vi "Write To FPGA.vi"(7 "Group.Rate":u32[](array[numeric]), 8 "error in (no error)":errorcluster, 9 "Changed?":bool[](array[boolean]), 10 "Values":dbl[](array[numeric]), 11 "FPGA Refs":T1 {"Data Type" format="%.0x"}) -> (0 "error out":errorcluster, 2 "Values out":dbl[](array[numeric]), 3 "FPGA Refs":T1 {"Data Type" format="%.0x"})   [LabVIEW 2019, in "Fuel Injector Analysis Addon Engine.lvlib"]
uses:
  Fuel Injector Analysis Addon Engine.lvlib
  Types/FPGA Refs.ctl
  Addon Shared/Types/FPGA Data Types.ctl
  <vilib>/Utility/error.llb/Error Cluster From Error Code.vi
  <vilib>/rvi/errors/niLvFpgaAdjustHostInterfaceError.vi
  <vilib>/rvi/interface/nirviReadWriteControl/nirviReadWriteControl.xnode
  <vilib>/rvi/interface/Simulation/niFpgaSimulationCallBeginRW.vi
  NiFpgaLv.dll
  Addon Shared/Fuel Injector Analysis Addon Shared.lvlib
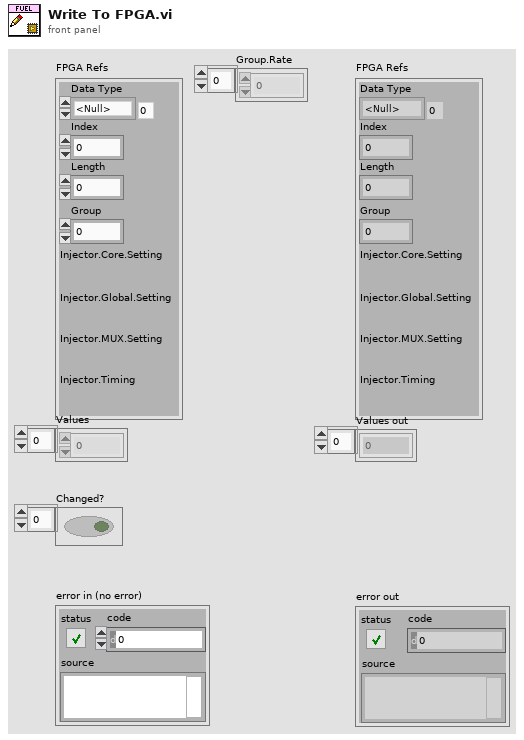
[diagram p1: front panel]
types:
  T1 = typedef "Fuel Injector Analysis Addon Engine.lvlib/FPGA Refs.ctl" = cluster{"Data Type":T2, "Index":i32, "Length":i32, "Group":i32, "Injector.Core.Setting":refnum<k20>, "Injector.Global.Setting":refnum<k20>, "Injector.MUX.Setting":refnum<k20>, "Injector.Timing":refnum<k20>}
  T2 = typedef "Fuel Injector Analysis Addon Shared.lvlib/FPGA Data Types.ctl" = enum8{"<Null>", "Injector.Core.Setting", "Injector.Global.Setting", "Injector.Mux.Setting", "Injector.Timing"}
  T3 = cluster{"Voltage Offset":fxp<+/-,32,8>, "Current Offset":fxp<+/-,32,8>}
  T4 = cluster{"Enable?":bool, "Initial Voltage Threshold":fxp<+/-,32,8>, "Event Dwell Limit":u16, "Voltage Gain":fxp<+/-,32,8>, "Current Gain":fxp<+/-,32,8>, "Filter Samples":u8, "Pretrigger Samples":u8, "Active Edge":bool}
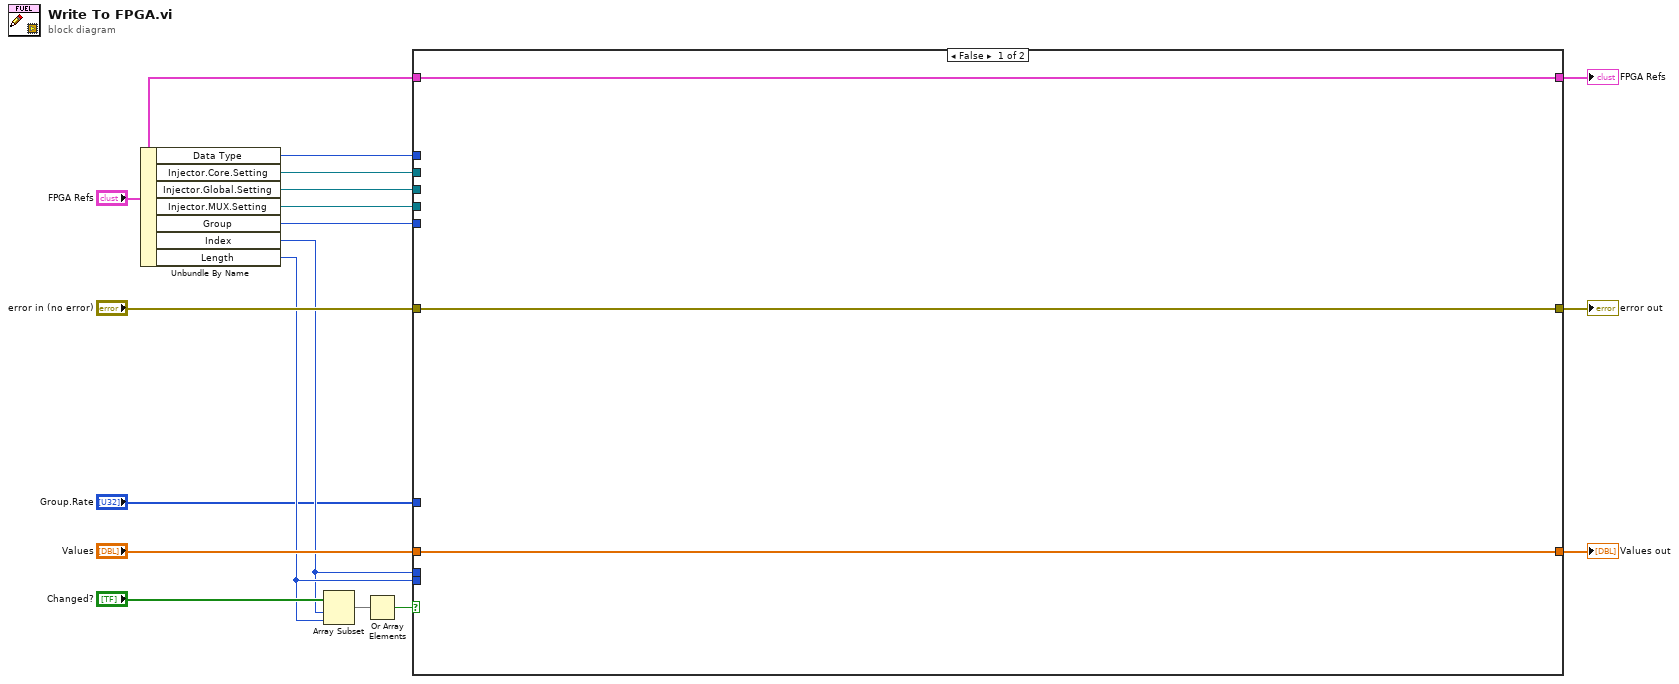
[diagram p0: block diagram]
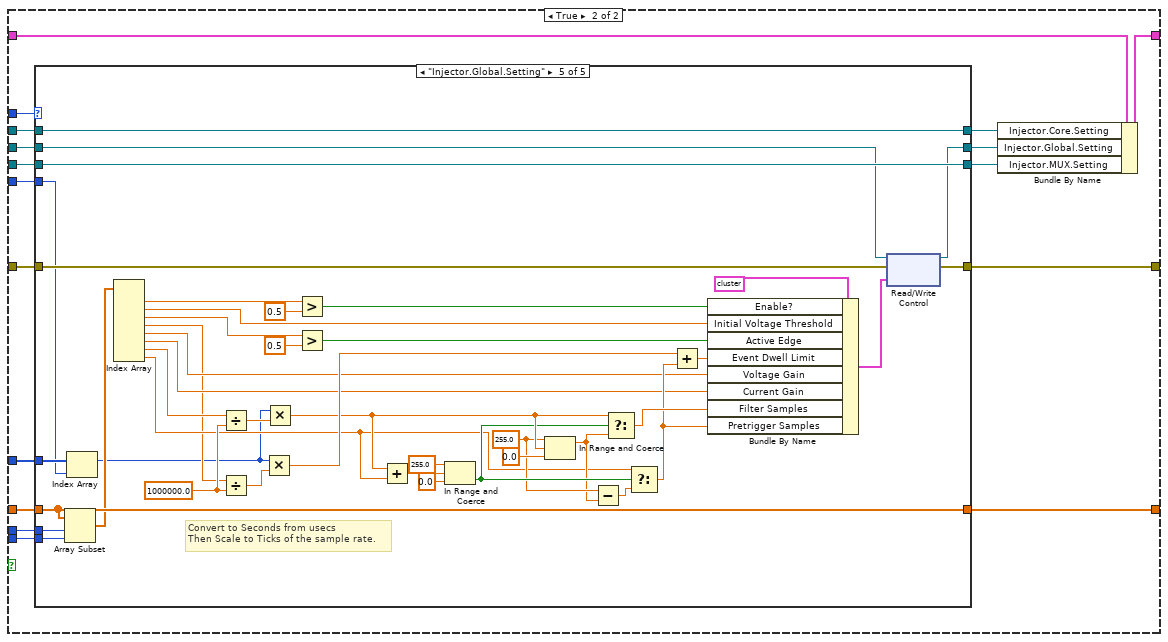
[diagram p2: hidden frame]
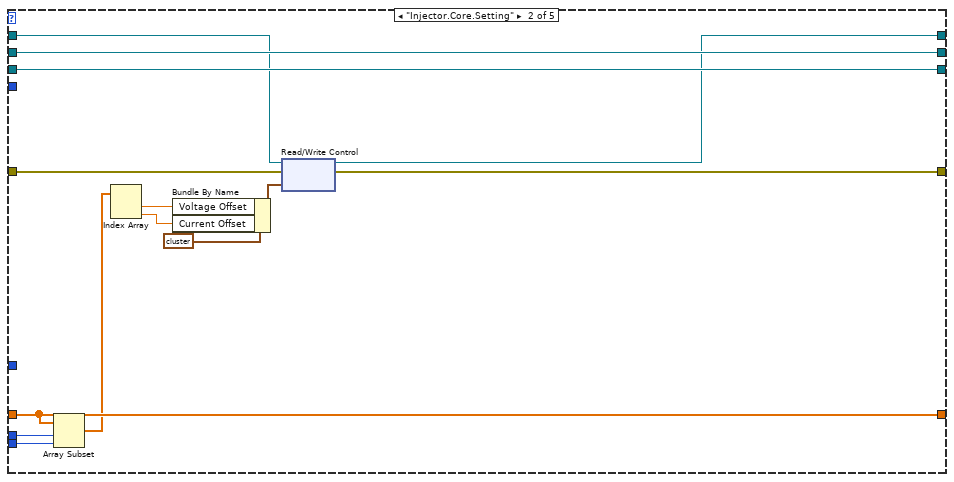
[diagram p4: hidden frame]
diagram:
  n1 = Unbundle By Name("FPGA Refs") -> ("Data Type"=w17:T2, "Injector.Core.Setting"=w8:refnum<k20>, "Injector.Global.Setting"=w12:refnum<k20>, "Injector.MUX.Setting"=w13:refnum<k20>, "Group"=w1:i32, "Index"=w3:i32, "Length"=w4:i32)
  n2 = Array Subset(array="Changed?", index=w3, length=w4) -> (w10:bool[])
  n3 = Or Array Elements(Boolean array=w10) -> (logical OR=w9:bool)
  n4 = case shown="False" w9 {
    tunnel: w17 -> [_ w37]
    tunnel: "error in (no error)" -> [w19 w36]
    tunnel: [w19 w35] -> w16
    tunnel: "FPGA Refs" -> [w20 w34]
    tunnel: [w20 w33] -> w5
    tunnel: [w18 w32] -> w15
    tunnel: "Values" -> [w18 w31]
    tunnel: w13 -> [_ w30]
    tunnel: w12 -> [_ w27]
    tunnel: w3 -> [_ w26]
    tunnel: w4 -> [_ w25]
    tunnel: w8 -> [_ w24]
    tunnel: "Group.Rate" -> [_ w22]
    tunnel: w1 -> [_ w21]
    frame False {
    }
    frame True {
      n5 = case shown="\"Injector.Global.Setting\"" w37 {
        tunnel: w36 -> [w42 w55 w59 w64 w109]
        tunnel: [w42 w54 w59 w64 w108] -> w35
        tunnel: [w41 w51 w60 w65 w105] -> w32
        tunnel: w31 -> [w41 w51 w60 w65 w105]
        tunnel: w25 -> [_ w52 _ _ w106]
        tunnel: w26 -> [_ w53 _ _ w107]
        tunnel: w30 -> [w40 w49 w57 w62 w103]
        tunnel: [w40 w49 w57 w62 w103] -> w29
        tunnel: [w39 w56 w61 w66 w98] -> w28
        tunnel: w27 -> [w39 w56 w61 w66 w99]
        tunnel: w24 -> [w38 w48 w58 w63 w100]
        tunnel: [w38 w47 w58 w63 w100] -> w23
        tunnel: w22 -> [_ _ _ _ w94]
        tunnel: w21 -> [_ _ _ _ w67]
        frame "<Null>", Default {
        }
        frame "Injector.Core.Setting" {
          n6 = Array Subset(array=w51, index=w53, length=w52) -> (w50:dbl[])
          n7 = Index Array(array=w50) -> (element #1=w44:dbl, element #2=w43:dbl)  [unwired: 2 in]
          n8 = Bundle By Name(cluster=T3 {"Voltage Offset"=0.0, "Current Offset"=0.0} ("Value"), "Voltage Offset"=w44, "Current Offset"=w43) -> (w45:T3)
          n9 = xnode "Read/Write Control"("FPGA VI Reference In"=w48, "error in"=w55, "Value"=w45) -> ("FPGA VI Reference Out"=w47:refnum<k20>, "error out"=w54:errorcluster)
        }
        frame "Injector.Mux.Setting" {
          # "DLE NOTE - Only Set in Init"
        }
        frame "Injector.Timing" {
          # "DLE NOTE - Only Set in Init"
        }
        frame "Injector.Global.Setting" {
          w82 = 255.0 ("upper limit")
          w93 = 1000000.0 ("y")
          # "Convert to Seconds from usecs\nThen Scale to Ticks of the sample rate."
          n10 = Array Subset(array=w105, index=w107, length=w106) -> (w104:dbl[])
          n11 = Index Array(array=w94, index=w67) -> (element=w68:u32)
          n12 = Index Array(array=w104) -> (element #1=w102:dbl, element #2=w101:dbl, element #3=w72:dbl, element #4=w74:dbl, element #5=w75:dbl, element #6=w76:dbl, element #7=w77:dbl, element #8=w78:dbl)  [unwired: 8 in]
          n13 = Divide(x=w77, y=w93) -> (x/y=w95:dbl)
          n14 = Divide(x=w74, y=w93) -> (x/y=w96:dbl)
          n15 = Multiply(x=w68, y=w96) -> (x*y=w88:dbl)
          n16 = Multiply(x=w68, y=w95) -> (x*y=w84:dbl)
          n17 = Greater?(x=w102, y=0.5 ("x")) -> (0:w71:bool)
          n18 = Greater?(x=w72, y=0.5 ("x")) -> (0:w70:bool)
          n19 = Add(x=w84, y=w78) -> (x+y=w92:dbl)
          n20 = In Range and Coerce(upper limit=255.0, x=w92, lower limit=0.0) -> (In Range?=w83:bool)  [unwired: 1 out]
          n21 = In Range and Coerce(upper limit=w82, x=w84, lower limit=0.0) -> (coerced(x)=w81:dbl)  [unwired: 1 out]
          n22 = Subtract(x=w82, y=w81) -> (x-y=w80:dbl)
          n23 = Select(t=w84, s=w83, f=w81) -> (s? t:f=w89:dbl)
          n24 = Select(t=w78, s=w83, f=w80) -> (s? t:f=w86:dbl)
          n25 = Add(x=w88, y=w86) -> (x+y=w87:dbl)
          n26 = Bundle By Name(cluster=T4 {"Enable?"=FALSE, "Initial Voltage Threshold"=0.0, "Event Dwell Limit"=0, "Voltage Gain"=0.0, "Current Gain"=0.0, "Filter Samples"=0, "Pretrigger Samples"=0, "Active Edge"=FALSE} ("Value"), "Enable?"=w71, "Initial Voltage Threshold"=w101, "Active Edge"=w70, "Event Dwell Limit"=w87, "Voltage Gain"=w75, "Current Gain"=w76, "Filter Samples"=w89, "Pretrigger Samples"=w86) -> (w69:T4)
          n27 = xnode "Read/Write Control"("FPGA VI Reference In"=w99, "error in"=w109, "Value"=w69) -> ("FPGA VI Reference Out"=w98:refnum<k20>, "error out"=w108:errorcluster)
        }
      }
      n28 = Bundle By Name(cluster=w34, "Injector.Core.Setting"=w23, "Injector.Global.Setting"=w28, "Injector.MUX.Setting"=w29) -> (w33:T1)
    }
  }
  "FPGA Refs" <- w5
  "error out" <- w16
  "Values out" <- w15
